vi "Excel Report - Insert Formulas in Spreadsheet.vi"() -> ()   [LabVIEW 2023]
doc: "This example shows how to insert formulas in an Excel workbook to analyze data."
uses:
  <vilib>/addons/_office/_wordsub.llb/font.ctl
  <vilib>/Utility/NIReport.llb/Report Type.ctl
  <vilib>/Utility/NIReport.llb/Append Numeric Table to Report (wrap).vi
  <vilib>/Utility/NIReport.llb/NI_report.lvclass
  <vilib>/Utility/NIReport.llb/Excel/NI_Excel.lvclass
  <vilib>/Utility/NIReport.llb/NI_ReportGenerationCore.lvlib
panel:
  in  "Total Sum Formula":string="=SUM(A11:J11)"
  in  "Sum of Column Formulas":string[](array[string])=["=SUM(A1:A10)", "=SUM(B1:B10)", "=SUM(C1:C10)", "=SUM(D1:D10)", "=SUM(E1:E10)", "=SUM(F1:F10)", "=SUM(G1:G10)", "=SUM(H1:H10)", "=SUM(I1:I10)", "=SUM(J1:J10)"] caption="Array Constant"
  # "Overview: This example shows how to insert formulas in an Excel workbook in order to analyze data.\nRequirements: Report Generation Toolkit, Microsoft Excel\nInstructions:\nRun the VI.\n\nNote: The formulas must be Excel formulas."
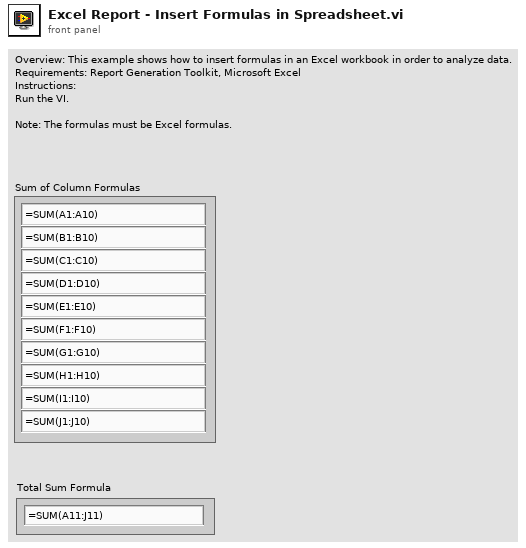
[diagram p1: front panel]
types:
  T1 = typedef "NI_ReportGenerationCore.lvlib/Report Type.ctl" = enum16{"HTML", "Word", "Excel"}
  T2 = typedef "font.ctl" = cluster{"font name":string, "font size":dbl, "bold":u16, "italic":u16, "underline":u16, "strike through":u16, "font color":u32}
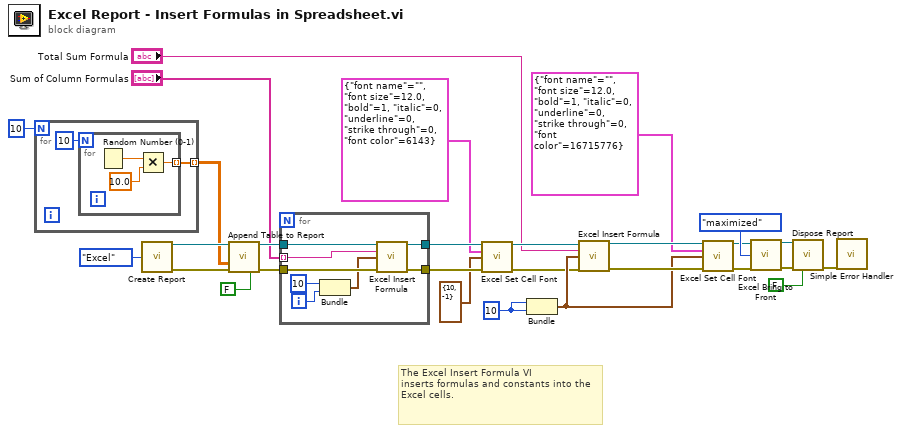
[diagram p0: block diagram]
diagram:
  w21 = 10
  # "The Excel Insert Formula VI \ninserts formulas and constants into the Excel cells."
  n1 = for {
    N: 10 -> [_]
    tunnel: [w30] -> w2 mode=indexing
    n2 = for {
      N: 10 ("dimension size") -> [_]
      tunnel: [w32] -> w30 mode=indexing
      n3 = Random Number (0-1)() -> (number: 0 to 1=w33:dbl)
      n4 = Multiply(x=w33, y=10.0) -> (x*y=w32:dbl)
    }
  }
  n5 = call <vilib>:"Create Report.vi"("report type"=Report_Type."Excel" ("Report Type")) -> ("report out"=w24:refnum<class "NI_report.lvclass">, "error out"=w25:errorcluster)  [unwired: 13 in]
  n6 = call-poly <vilib>:"Append Table to Report.vi"("report in"=w24, "numerical data"=w2, "error in (no error)"=w25, "show grid lines"=FALSE) -> ("report out"=w27:refnum<class "NI_report.lvclass">, "error out"=w28:errorcluster)  [unwired: 8 in, 2 out]
  n7 = for {
    tunnel: w28 -> [w41]
    tunnel: w27 -> [w40]
    tunnel: [w36] -> w18
    tunnel: [w35] -> w17
    tunnel: "Sum of Column Formulas" -> [w34] mode=indexing
    i -> [w38]
    n8 = Bundle("Row"=10, w38) -> (w37:cluster{"Row":i32, i32})  [unwired: 1 in]
    n9 = call <vilib>:"Excel Insert Formula.vi"("report in"=w40, "formula"=w34, "start (0, 0)"=w37, "error in (no error)"=w41) -> ("report out"=w35:refnum<class "NI_report.lvclass">, "error out"=w36:errorcluster)  [unwired: 10 in]
  }
  n10 = call <vilib>:"Excel Set Cell Font.vi"("report in"=w17, "font"=T2 {"font name"="", "font size"=12.0, "bold"=1, "italic"=0, "underline"=0, "strike through"=0, "font color"=6143}, "start (-1, -1)"=cluster{"row":i32, "column":i32} {"row"=10, "column"=-1}, "error in (no error)"=w18) -> ("report out"=w15:refnum<class "NI_report.lvclass">, "error out"=w16:errorcluster)  [unwired: 10 in]
  n11 = Bundle(w21, w21) -> (w20:cluster{i32, i32})  [unwired: 1 in]
  n12 = call <vilib>:"Excel Insert Formula.vi"("report in"=w15, "formula"="Total Sum Formula", "start (0, 0)"=w20, "error in (no error)"=w16) -> ("report out"=w23:refnum<class "NI_report.lvclass">, "error out"=w26:errorcluster)  [unwired: 10 in]
  n13 = call <vilib>:"Excel Set Cell Font.vi"("report in"=w23, "font"=T2 {"font name"="", "font size"=12.0, "bold"=1, "italic"=0, "underline"=0, "strike through"=0, "font color"=16715776}, "start (-1, -1)"=w20, "error in (no error)"=w26) -> ("report out"=w10:refnum<class "NI_report.lvclass">, "error out"=w11:errorcluster)  [unwired: 10 in]
  n14 = call <vilib>:"Excel Bring to Front.vi"("report in"=w10, "window state (maximized)"=enum16{"maximized", "minimized", "normal"}."maximized", "error in (no error)"=w11) -> ("report out"=w9:refnum<class "NI_report.lvclass">, "error out"=w8:errorcluster)  [unwired: 11 in]
  n15 = call-dynamic "Dispose Report.vi"("report in"=w9, "error in (no error)"=w8, "close report? (T)"=FALSE ("Close Report? (T)")) -> ("error out"=w7:errorcluster)  [unwired: 12 in]
  n16 = call <vilib>:"Simple Error Handler.vi"("error in (no error)"=w7) -> ()  [unwired: 4 in, 5 out]
